vi "Level_Function.vi"(7 "Level":bool, 8 "lower Limit":dbl=720.0 format="%#_13g", 9 "upper limit":dbl) -> (3 "Level":bool=TRUE)   [LabVIEW 2014]
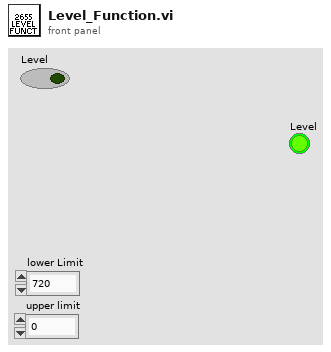
[diagram p1: front panel]
types:
  T1 = typedef "WPI_EncoderDevRef.ctl" = cluster{"DevStatus":errorcluster, "EncoderIndex":T2, "CounterIndex":T3, "DistancePerCount":dbl, "Decoding Type":T4}
  T2 = typedef "FPGA_EncoderIdx.ctl" = enum8{"Enc 0", "Enc 1", "Enc 2", "Enc 3", "Enc 4", "Enc 5", "Enc 6", "Enc 7", "Invalid"}
  T3 = typedef "FPGA_CounterCtrSystemIndex.ctl" = enum8{"Ctr 0", "Ctr 1", "Ctr 2", "Ctr 3", "Ctr 4", "Ctr 5", "Ctr 6", "Ctr 7", "Invalid"}
  T4 = typedef "WPI_EncoderType.ctl" = enum16{"1x", "2x", "4x"}
  T5 = typedef "WPI_MotorControlDeviceRef.ctl" = cluster{"DeviceStatus":errorcluster, "Type":T6, "PWM":cluster{"Controller":T7, "PWM Channel":T8, "DeadBand":T9}, "CAN":cluster{"Device Number":u8, "Control Mode":T10, "Semaphore":T11, "Max Vout":dbl, "TalonSRX Control Mode":T12}, "Invert":bool, "TransformRef":T13, "InvTransformRef":T13}
  T6 = typedef "WPI_MotorControlType.ctl" = enum16{"PWM", "CAN", "CANTalonSRX"}
  T7 = typedef "FPGA_TypedefDigitalModule.ctl" = enum16{"Controller 1"}
  T8 = typedef "FPGA_DIOPWMChannel.ctl" = enum8{"PWM 0", "PWM 1", "PWM 2", "PWM 3", "PWM 4", "PWM 5", "PWM 6", "PWM 7", "PWM 8", "PWM 9", "PWM MXP 0", "PWM MXP 1", "PWM MXP 2", "PWM MXP 3", "PWM MXP 4", "PWM MXP 5", "PWM MXP 6", "PWM MXP 7", "PWM MXP 8", "PWM MXP 9", "Invalid"}
  T9 = typedef "WPI_PWMDeadband.ctl" = cluster{"Name":string, "maxPositivePwm":i32, "minPositivePwm":i32, "centerPwm":i32, "maxNegativePwm":i32, "minNegativePwm":i32, "angularRange":u16}
  T10 = typedef "WPI_CANJaguar_ControlMode.ctl" = enum8{"Percent VBus", "Current", "Speed", "Position", "Voltage"}
  T11 = typedef "Semaphore RefNum" = refnum<k1>
  T12 = typedef "WPI_CANTalonSRX_APIControlMode.ctl" = enum8{"Percent VBus", "Speed", "Position", "Slave", "Unchanged / Invalid"}
  T13 = typedef "WPI_PWMTransform_ConPane.ctl" = refnum<vi>
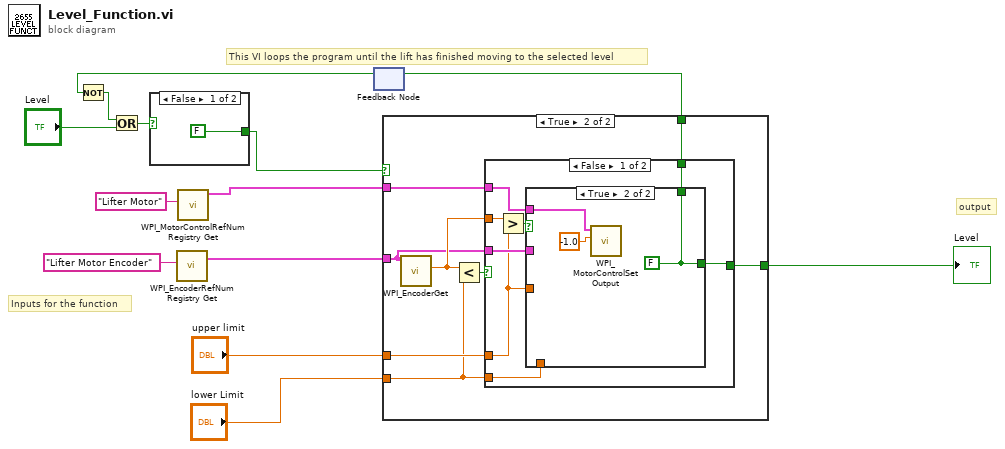
[diagram p0: block diagram]
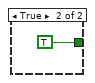
[diagram p2: hidden frame]
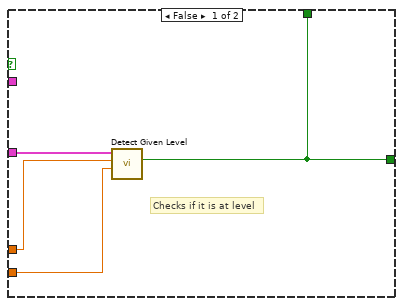
[diagram p3: hidden frame]
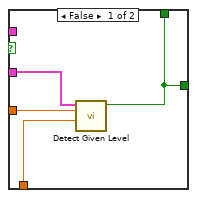
[diagram p4: hidden frame]
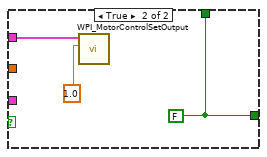
[diagram p5: hidden frame]
diagram:
  # "output"
  # "Inputs for the function"
  # "This VI loops the program until the lift has finished moving to the selected level"
  n1 = call <vilib>:"WPI_EncoderRefNum Registry Get.vi"("refnum name"="Lifter Motor Encoder") -> ("EncoderDevRef"=w1:T1)  [unwired: 9 in, 1 out]
  n2 = call <vilib>:"WPI_MotorControlRefNum Registry Get.vi"("refnum name"="Lifter Motor") -> ("MotorControlDevRef"=w3:T5)  [unwired: 9 in, 1 out]
  n3 = feedback #1() -> (w5:bool)  [unwired: 1 in]
  n4 = Not(x=w5) -> (.not. x?=w6:bool)
  n5 = Or(x=w6, y="Level") -> (x .or. y?=w8:bool)
  n6 = case shown="False" w8 {
    tunnel: [FALSE TRUE] -> w7
    frame False {
    }
    frame True {
    }
  }
  n7 = case shown="True" w7 {
    tunnel: [w16 w26] -> w13
    tunnel: w1 -> [w19 w24]
    tunnel: w3 -> [_ w23]
    tunnel: "lower Limit" -> [w17 w21]
    tunnel: "upper limit" -> [w18 w22]
    tunnel: [w16 w20] -> w9
    frame False {
      # "Checks if it is at level"
      n8 = call "Detect Given Level.vi"("lower limit"=w17, "upper limit"=w18, "EncoderDevRef"=w19) -> ("At level"=w16:bool)  [unwired: 8 in]
    }
    frame True {
      n9 = call <vilib>:"WPI_EncoderGet.vi"("EncoderDevRef"=w24) -> ("Distance"=w25:dbl)  [unwired: 5 in, 5 out]
      n10 = Less?(x=w25, y=w21) -> (x < y?=w27:bool)
      n11 = case shown="False" w27 {
        tunnel: [w33 w43] -> w26
        tunnel: w25 -> [w35 _]
        tunnel: w24 -> [w32 _]
        tunnel: w23 -> [w31 w44]
        tunnel: w22 -> [w30 _]
        tunnel: w21 -> [w28 _]
        tunnel: [w29 w43] -> w20
        frame False {
          n12 = Greater?(x=w35, y=w30) -> (0:w34:bool)
          n13 = case shown="True" w34 {
            tunnel: [w36 w40] -> w33
            tunnel: w32 -> [w39 _]
            tunnel: w31 -> [_ w41]
            tunnel: w30 -> [w38 _]
            tunnel: w28 -> [w37 _]
            tunnel: [w36 w40] -> w29
            frame False {
              n14 = call "Detect Given Level.vi"("lower limit"=w37, "upper limit"=w38, "EncoderDevRef"=w39) -> ("At level"=w36:bool)  [unwired: 8 in]
            }
            frame True {
              w40 = FALSE
              n15 = call <vilib>:"WPI_MotorControlSetOutput.vi"("Output"=-1.0, "MotorControlDevRef"=w41) -> ()  [unwired: 7 in, 3 out]
            }
          }
        }
        frame True {
          w43 = FALSE
          n16 = call <vilib>:"WPI_MotorControlSetOutput.vi"("Output"=1.0, "MotorControlDevRef"=w44) -> ()  [unwired: 7 in, 3 out]
        }
      }
    }
  }
  "Level" <- w13
  n17 = feedback-in #1(w9) -> ()
